vi "Obtain Groups.vi"(8 "error in (no error)":errorcluster, 11 "GenericGuiAO in":refnum<class "GenericGuiAO.lvclass">) -> (0 "error out":errorcluster, 3 "GenericGuiAO out":refnum<class "GenericGuiAO.lvclass">)   [LabVIEW 2020, in "VolatusDAQGenericGUI.lvlib" / "GenericGuiAO.lvclass"]
uses:
  GenericGuiAO.lvclass
  GenericGuiAO.lvclass/GenericGuiAO.ctl
  Volatus/Module/Module.lvclass
  C:/dev/lv20CE/relink/lv-volatus/Volatus/Module/Module.lvclass
  C:/dev/lv20CE/relink/lv-volatus/VolatusDAQGenericGUI/GenericGuiAO/GenericGuiAO.lvclass
  VolatusDAQGenericGUI.lvlib
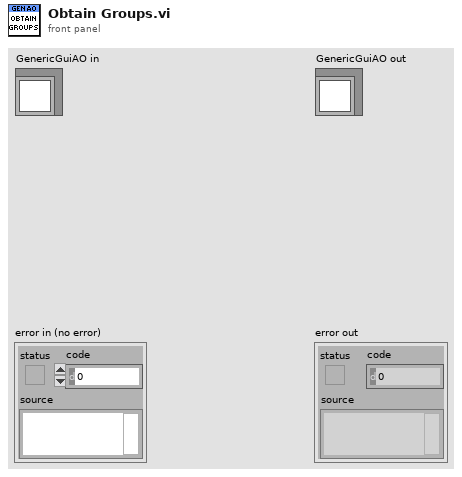
[diagram p1: front panel]
types:
  T1 = typedef "VolatusDAQGenericGUI.lvlib/Group Info.ctl" = cluster{"Group":refnum<class "Group.lvclass">, "Channel Names":string[], "Resources":string[], "Node":string, "Task":string}
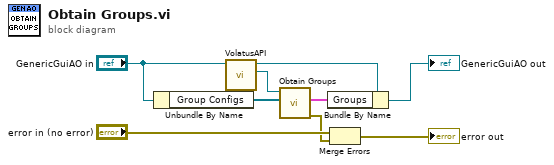
[diagram p0: block diagram]
diagram:
  n1 = Unbundle By Name("GenericGuiAO in") -> ("Group Configs"=w4:refnum<class "Group.lvclass">[])
  n2 = call "VolatusAPI.vi"("Module in"="GenericGuiAO in") -> ("VolatusAPI"=w3:refnum<class "VolatusAPI.lvclass">, "Module out"=w9:refnum<class "GenericGuiAO.lvclass">)  [unwired: 9 in]
  n3 = call "Obtain Groups.vi"("Group Configs"=w4, "VolatusAPI"=w3) -> ("error out"=w2:errorcluster, "Groups"=w1:T1[])  [unwired: 8 in]
  n4 = Bundle By Name(cluster=w9, "Groups"=w1) -> (→"GenericGuiAO out":refnum<class "GenericGuiAO.lvclass">)
  n5 = Merge Errors("error in (no error)", w2) -> (→"error out":errorcluster)
